vi "Project Path.vi"(10 "Project:Active Project":refnum<vi>) -> (2 "Project Path":path)   [LabVIEW 2025, in "_Shared.lvlib"]
uses:
  _Shared.lvlib
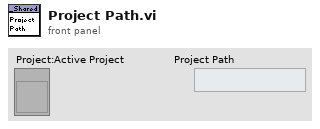
[diagram p1: front panel]
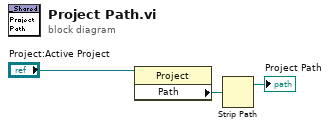
[diagram p0: block diagram]
diagram:
  n1 = property class="Project"(reference="Project:Active Project") -> ("Path"=w3:path)  [unwired: 1 in, 2 out]
  n2 = Strip Path(path=w3) -> (stripped path=→"Project Path":path)  [unwired: 1 out]
